vi "Configure Multi Eval Meas LO Leakage Limit.vi"(7 "LO Leakage (Off)":bool, 8 "error in (no error)":errorcluster, 9 "LO Leakage (0)":dbl format="%^.3e", 10 "Instance (1)":i32=1, 11 "VISA resource name":refnum<visa-resource-name>) -> (0 "error out":errorcluster, 3 "VISA resource name out":refnum<visa-resource-name>)   [LabVIEW 2015, in "Rohde&Schwarz CMP LR WPAN Measurement.lvlib"]
doc: "Defines upper limit for the LO leakage value.\n\nOrder of parameters:\n<LO_Leakage> - Local scillator leakage\n<LO_Leakage_Enb> - Disables or enables the limit check for LO leakage.\n\nAttribute:\n-\n\nRemote-control command:\nCONFigure:WPAN:MEAS<i>:MEValuation:LIMit:LLEakage"
uses:
  <instrlib>/Rohde&Schwarz CMP LR WPAN Measurement/Rohde&Schwarz CMP LR WPAN Measurement.lvlib
  <instrlib>/Rohde&Schwarz CMP LR WPAN Measurement/Private/rsidr_core.llb/rsidr_core.lvlib
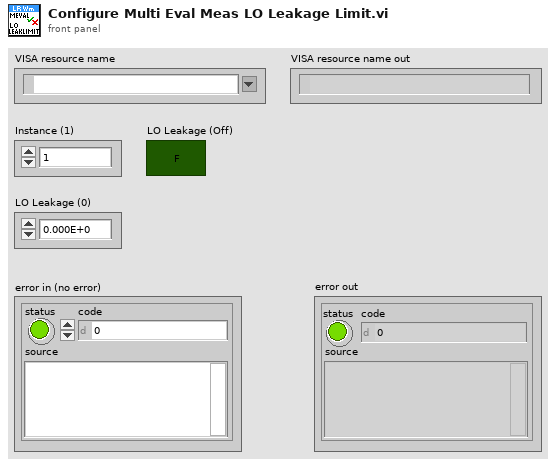
[diagram p1: front panel]
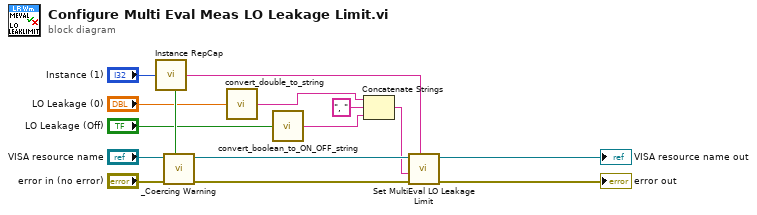
[diagram p0: block diagram]
diagram:
  n1 = call <instrlib>:"Instance RepCap.vi"("Instance In"="Instance (1)") -> ("In Range?"=w15:bool, "RepCap Identifier Out"=w13:string)  [unwired: 1 in]
  n2 = call <instrlib>:"_Coercing Warning.vi"("In Range?"=w15, "error in (no error)"="error in (no error)", "VISA resource name"="VISA resource name") -> ("error out"=w6:errorcluster, "VISA resource name out"=w5:refnum<visa-resource-name>)  [unwired: 7 in]
  n3 = call <instrlib>:"convert_double_to_string.vi"("double in"="LO Leakage (0)") -> ("string out"=w11:string)  [unwired: 4 in]
  n4 = call <instrlib>:"convert_boolean_to_ON_OFF_string.vi"("boolean value in"="LO Leakage (Off)") -> ("string value out"=w9:string)  [unwired: 4 in]
  n5 = Concatenate Strings(w11, ", " ("string"), w9) -> (w2:string)
  n6 = call "Set MultiEval LO Leakage Limit"("Repeated Capabilities"=w13, "error in (no error)"=w6, "MultiEval LO Leakage Limit ()"=w2, "instrument handle"=w5) -> ("error out"=→"error out":errorcluster, "instrument handle out"=→"VISA resource name out":refnum<visa-resource-name>)  [unwired: 6 in]
